vi "Set_IP_Simulation_Direction.vi"(8 "error in (no error)":errorcluster, 9 "Cellular Tech":string="ip_simulation", 10 "value":string(combo), 11 "Base Station":T1) -> (0 "error out":errorcluster, 3 "Output String":string)   [LabVIEW 2021]
uses:
  Controls/Base_Station_Emulator.ctl
  Controls/TCP_FGV.ctl
panel:
  # "0 - dl\n1- ul\n2 - dl_ul"
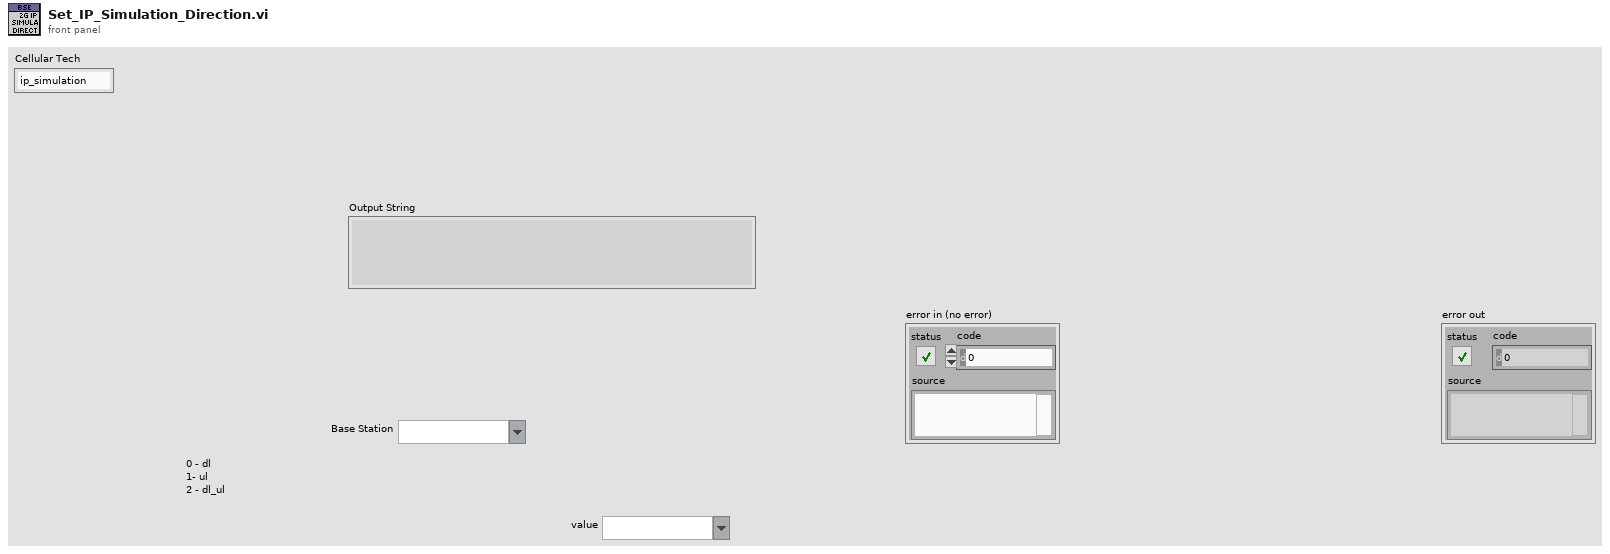
[diagram p1: front panel]
types:
  T1 = typedef "Base_Station_Emulator.ctl" = string
  T2 = typedef "TCP_FGV.ctl" = enum16{"Open", "Read", "Write", "Close"}
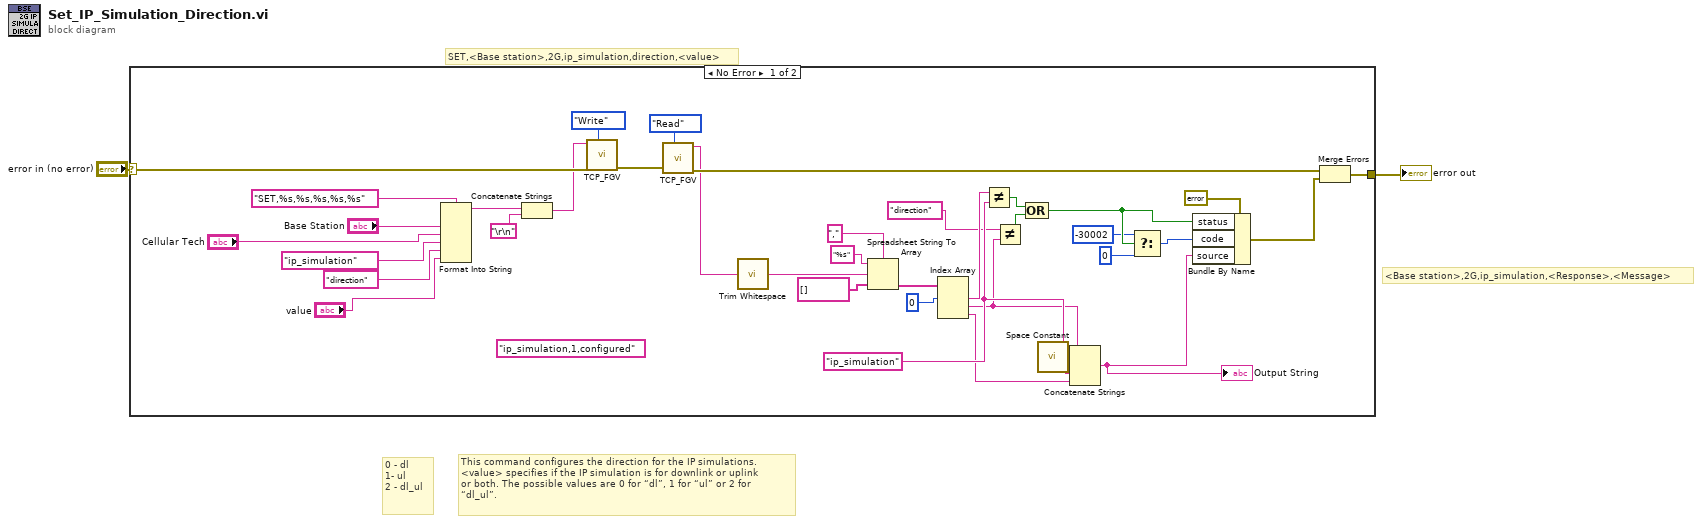
[diagram p0: block diagram]
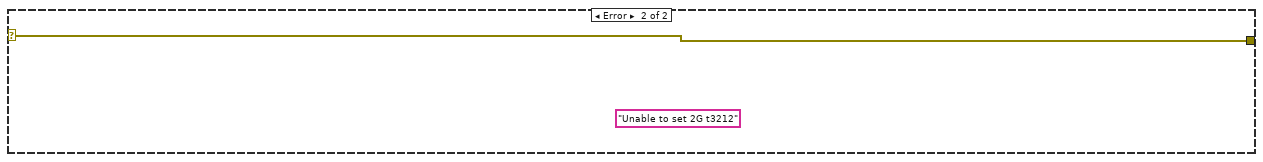
[diagram p2: hidden frame]
diagram:
  # "0 - dl\n1- ul\n2 - dl_ul"
  # "<Base station>,2G,ip_simulation,<Response>,<Message>"
  # "This command configures the direction for the IP simulations.  \n<value> specifies if the IP simulation is for downlink or uplink \nor both. The possible values are 0 for “dl”, 1 for “ul” or 2 for  \n“dl_ul”."
  # "SET,<Base station>,2G,ip_simulation,direction,<value>"
  n1 = case shown="No Error" "error in (no error)" {
    selector: "error in (no error)" -> [w36 w40]
    tunnel: [w21 w40] -> w1
    frame No Error {
      (unwired) "ip_simulation,1,configured" ("format string")
      w13 = "ip_simulation" ("format string")
      n2 = Format Into String(format string="SET,%s,%s,%s,%s,%s", "Base Station", "Cellular Tech", "ip_simulation", "direction", "value") -> (resulting string=w16:string)  [unwired: 2 in, 1 out]
      n3 = Concatenate Strings(w16, "\r\n") -> (w15:string)
      n4 = call "TCP_FGV.vi"("Command"=w15, "error in (no error)"=w36, "Operation"=TCP_FGV."Write") -> ("error out"=w22:errorcluster)  [unwired: 6 in, 1 out]
      n5 = call "TCP_FGV.vi"("error in (no error)"=w22, "Operation"=TCP_FGV."Read") -> ("Data Out"=w10:string, "error out"=w24:errorcluster)  [unwired: 7 in]
      n6 = call <vilib>:"Trim Whitespace.vi"("string"=w10) -> ("trimmed string"=w33:string)  [unwired: 1 in]
      n7 = Spreadsheet String To Array(delimiter (Tab)=",", format string="%s", spreadsheet string=w33, array type (2D Dbl)=string[] []) -> (array=w32:string[])
      n8 = Index Array(array=w32, index #1=0 ("index")) -> (element #1=w25:string, element #2=w6:string, element #3=w11:string)  [unwired: 2 in]
      n9 = Not Equal?(x=w25, y=w13) -> (x != y?=w8:bool)
      n10 = Not Equal?(x="direction", y=w6) -> (x != y?=w7:bool)
      n11 = Compound Arithmetic op=OR(w8, w7) -> (w34:bool)
      n12 = call <vilib>:"Space Constant.vi"() -> ("String"=w12:string)
      n13 = Concatenate Strings(w13, w12, w6, w12, w11) -> (w20:string)
      "Output String" <- w20
      n14 = Select(t=-30002 ("code"), s=w34, f=0 ("code")) -> (s? t:f=w35:i32)
      n15 = Bundle By Name(cluster=errorcluster {"status"=FALSE, "code"=0, "source"=""} ("error constant"), "status"=w34, "code"=w35, "source"=w20) -> (w23:errorcluster)
      n16 = Merge Errors(w24, w23) -> (w21:errorcluster)
    }
    frame Error {
      (unwired) "Unable to set 2G t3212" ("source")
    }
  }
  "error out" <- w1
